vi "LCD Retarder.vi"(8 "error in":errorcluster, 11 "LCD In":refnum<class "LCD Retarder.lvclass">) -> (0 "errorOUT":errorcluster, 3 "LCD out":refnum<class "LCD Retarder.lvclass">)   [LabVIEW 2012, in "LCD Retarder.lvclass"]
uses:
  LCD Retarder.lvclass
  LCD Retarder.lvclass/LCD Retarder.ctl
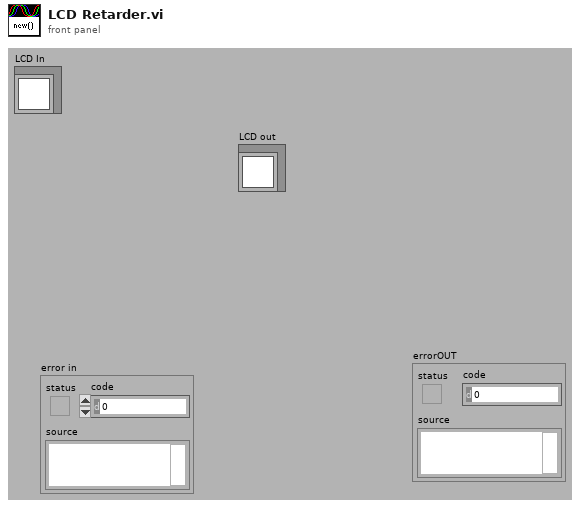
[diagram p1: front panel]
types:
  T1 = cluster{"Device Handle":u32, "Pipe 0 Handle":u32, "Pipe 1 Handle":u32}[]
  T2 = cluster{"Device Handle":u32, "Pipe 0 Handle":u32, "Pipe 1 Handle":u32}
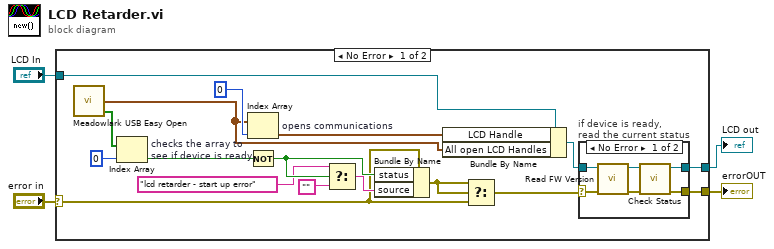
[diagram p0: block diagram]
diagram:
  n1 = case shown="No Error" "error in" {
    selector: "error in" -> [w5 w30]
    tunnel: [w21 w31] -> w4
    tunnel: "LCD In" -> [w20 w31]
    tunnel: [w18 w30] -> w2
    frame No Error {
      n2 = call "Meadowlark USB Easy Open.vi"() -> ("Device Opened Array"=w13:bool[], "USB Device and Pipes Array"=w8:T1)  [unwired: 1 out]
      n3 = Index Array "checks the array to\nsee if device is ready"(array=w13, index=0) -> (element=w19:bool)
      n4 = Index Array "opens communications"(array=w8, index=0) -> (element=w9:T2)
      n5 = Not(x=w19) -> (.not. x?=w16:bool)
      n6 = Select(t="lcd retarder - start up error", s=w16, f="") -> (s? t:f=w17:string)
      n7 = Bundle By Name(cluster=w5, "status"=w16, "source"=w17) -> (w7:errorcluster)
      n8 = Bundle By Name(cluster=w20, "LCD Handle"=w9, "All open LCD Handles"=w8) -> (w10:refnum<class "LCD Retarder.lvclass">)
      n9 = Select(t=w7, s=w7, f=w5) -> (s? t:f=w6:errorcluster)
      n10 = case "if device is ready,\nread the current status" shown="No Error" w6 {
        selector: w6 -> [w26 w29]
        tunnel: [w22 w29] -> w18
        tunnel: w10 -> [w27 w28]
        tunnel: [w24 w28] -> w21
        frame No Error {
          n11 = call "Read FW Version.vi"("errorIN"=w26, "LCD in"=w27) -> ("error out"=w23:errorcluster, "LCD out"=w25:refnum<class "LCD Retarder.lvclass">)  [unwired: 8 out]
          n12 = call-dynamic "Check Status.vi"("error in (no error)"=w23, "LCD Retarder in"=w25) -> ("error out"=w22:errorcluster, "LCD Retarder out"=w24:refnum<class "LCD Retarder.lvclass">)  [unwired: 6 in, 2 out]
        }
        frame Error {
        }
      }
    }
    frame Error {
    }
  }
  "LCD out" <- w4
  "errorOUT" <- w2
